vi "GET.vi"() -> ()   [LabVIEW 2021]
uses:
  <vilib>/httpClient/LabVIEWHTTPClient.lvlib
panel:
  out "headers":string
  out "body":string
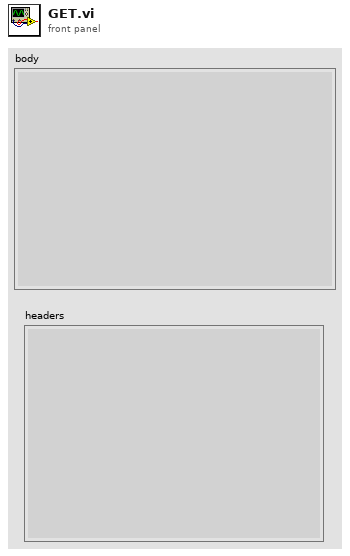
[diagram p1: front panel]
types:
  T1 = typedef "LabVIEWHTTPClient.lvlib/ClientHandle.ctl" = refnum<k1>
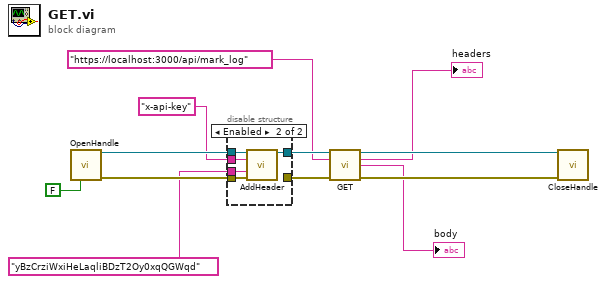
[diagram p0: block diagram]
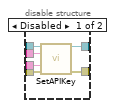
[diagram p2: hidden frame]
diagram:
  n1 = call <vilib>:"OpenHandle.vi"("verify server(true)"=FALSE) -> ("client handle out"=w12:T1, "error out"=w11:errorcluster)  [unwired: 13 in]
  n2 = disable-structure shown="Enabled" {
    disable-tunnel: w12 -> [w18 w22]
    disable-tunnel: w11 -> [w17 w19]
    disable-tunnel: [w16 w23] -> w10
    disable-tunnel: [w15 _] -> w9
    disable-tunnel: "x-api-key" ("access id") -> [w14 w21]
    disable-tunnel: "yBzCrziWxiHeLaqliBDzT2Oy0xqQGWqd" ("secret id") -> [w13 w20]
    frame Disabled {
      n3 = call <vilib>:"SetAPIKey.vi"("client handle"=w18, "access id"=w14, "secret id"=w13, "error in (no error)"=w17) -> ("client handle out"=w16:T1, "error out"=w15:errorcluster)  [unwired: 10 in]
    }
    frame Enabled {
      n4 = call <vilib>:"AddHeader.vi"("client handle"=w22, "header"=w21, "value"=w20, "error in (no error)"=w19) -> ("client handle out"=w23:T1)  [unwired: 10 in, 1 out]
    }
  }
  n5 = call <vilib>:"GET.vi"("client handle"=w10, "url"="https://localhost:3000/api/mark_log", "error in (no error)"=w9) -> ("client handle out"=w8:T1, "headers"=→"headers":string, "body"=→"body":string, "error out"=w7:errorcluster)  [unwired: 9 in]
  n6 = call <vilib>:"CloseHandle.vi"("client handle"=w8, "error in (no error)"=w7) -> ()  [unwired: 13 in, 1 out]
